vi "get_ACS_status.vi"() -> ()   [LabVIEW 2018]
uses:
  S4GEI/S4GEI/RxTx/RxTx.lvclass
  <vilib>/addons/zeromq/socket_type.ctl
  <vilib>/addons/zeromq/socket_options.ctl
  <vilib>/addons/zeromq/zmq_socket.lvclass
  <vilib>/addons/zeromq/zmq_context.lvclass
  <vilib>/addons/zeromq/zeromq.lvlib
panel:
  in  "RxTx in":refnum<class "RxTx.lvclass">
  in  "Stop Button":bool
  out "error out":errorcluster
  out "error out 3":errorcluster
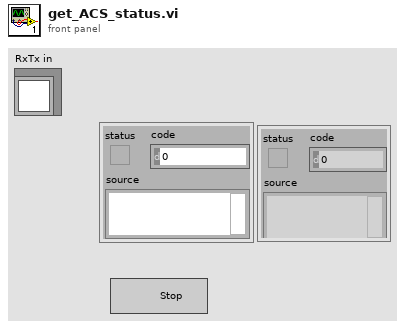
[diagram p1: front panel]
types:
  T1 = typedef "zeromq.lvlib/socket_options.ctl" = enum8{"NONE", "ZMQ_HWM", "<2>", "ZMQ_SWAP", "ZMQ_AFFINITY", "ZMQ_ROUTING_ID", "ZMQ_SUBSCRIBE", "ZMQ_UNSUBSCRIBE", "ZMQ_RATE", "ZMQ_RECOVERY_IVL", "ZMQ_MCAST_LOOP", "ZMQ_SNDBUF", "ZMQ_RCVBUF", "ZMQ_RCVMORE", "ZMQ_FD", "ZMQ_EVENTS", "ZMQ_TYPE", "ZMQ_LINGER", "ZMQ_RECONNECT_IVL", "ZMQ_BACKLOG", "ZMQ_RECOVERY_IVL_MSEC", "ZMQ_RECONNECT_IVL_MAX", "ZMQ_MAXMSGSIZE", "ZMQ_SNDHWM", "ZMQ_RCVHWM", "ZMQ_MULTICAST_HOPS", "<26>", "ZMQ_RCVTIMEO", "ZMQ_SNDTIMEO", "<29>", "<30>", "ZMQ_IPV4ONLY", "ZMQ_LAST_ENDPOINT", "ZMQ_ROUTER_MANDATORY", "ZMQ_TCP_KEEPALIVE", "ZMQ_TCP_KEEPALIVE_CNT", "ZMQ_TCP_KEEPALIVE_IDLE", "ZMQ_TCP_KEEPALIVE_INTVL", "ZMQ_TCP_ACCEPT_FILTER", "ZMQ_IMMEDIATE", "ZMQ_XPUB_VERBOSE", "ZMQ_ROUTER_RAW", "ZMQ_IPV6", "ZMQ_MECHANISM", "ZMQ_PLAIN_SERVER", "ZMQ_PLAIN_USERNAME", "ZMQ_PLAIN_PASSWORD", "ZMQ_CURVE_SERVER", "ZMQ_CURVE_PUBLICKEY", "ZMQ_CURVE_SECRETKEY", "ZMQ_CURVE_SERVERKEY", "ZMQ_PROBE_ROUTER", "ZMQ_REQ_CORRELATE", "ZMQ_REQ_RELAXED", "ZMQ_CONFLATE", "ZMQ_ZAP_DOMAIN", "ZMQ_ROUTER_HANDOVER", "ZMQ_TOS", "ZMQ_IPC_FILTER_PID", "ZMQ_IPC_FILTER_UID", "ZMQ_IPC_FILTER_GID", "ZMQ_CONNECT_ROUTING_ID", "ZMQ_GSSAPI_SERVER", "ZMQ_GSSAPI_PRINCIPAL", "ZMQ_GSSAPI_SERVICE_PRINCIPAL", "ZMQ_GSSAPI_PLAINTEXT", "ZMQ_HANDSHAKE_IVL", "<67>", "ZMQ_SOCKS_PROXY", "ZMQ_XPUB_NODROP", "ZMQ_BLOCKY", "ZMQ_XPUB_MANUAL", "ZMQ_XPUB_WELCOME_MSG", "ZMQ_STREAM_NOTIFY", "ZMQ_INVERT_MATCHING", "ZMQ_HEARTBEAT_IVL", "ZMQ_HEARTBEAT_TTL", "ZMQ_HEARTBEAT_TIMEOUT", "ZMQ_XPUB_VERBOSER", "ZMQ_CONNECT_TIMEOUT", "ZMQ_TCP_MAXRT", "ZMQ_THREAD_SAFE", "<82>", "<83>", "ZMQ_MULTICAST_MAXTPDU", "ZMQ_VMCI_BUFFER_SIZE", "ZMQ_VMCI_BUFFER_MIN_SIZE", "ZMQ_VMCI_BUFFER_MAX_SIZE", "ZMQ_VMCI_CONNECT_TIMEOUT", "ZMQ_USE_FD", "ZMQ_GSSAPI_PRINCIPAL_NAMETYPE", "ZMQ_GSSAPI_SERVICE_PRINCIPAL_NAMETYPE", "ZMQ_BINDTODEVICE", "ZMQ_ZAP_ENFORCE_DOMAIN", "ZMQ_LOOPBACK_FASTPATH", "ZMQ_METADATA", "ZMQ_MULTICAST_LOOP", "ZMQ_ROUTER_NOTIFY"}
  T2 = typedef "zeromq.lvlib/socket_type.ctl" = enum8{"ZMQ_PAIR", "ZMQ_PUB", "ZMQ_SUB", "ZMQ_REQ", "ZMQ_REP", "ZMQ_DEALER", "ZMQ_ROUTER", "ZMQ_PULL", "ZMQ_PUSH", "ZMQ_XPUB", "ZMQ_XSUB", "ZMQ_STREAM", "ZMQ_SERVER", "ZMQ_CLIENT", "ZMQ_RADIO", "ZMQ_DISH", "ZMQ_GATHER", "ZMQ_SCATTER", "ZMQ_DGRAM"}
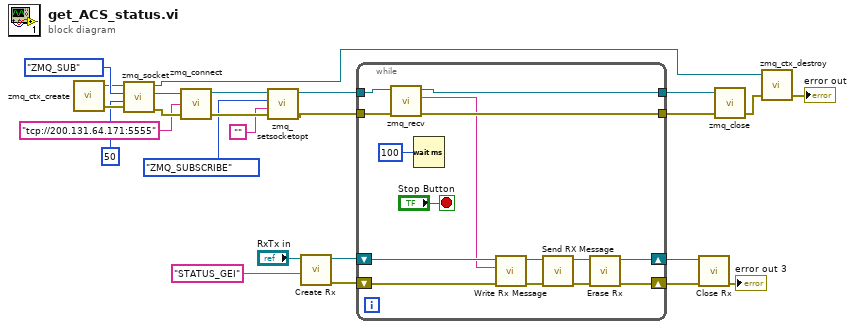
[diagram p0: block diagram]
diagram:
  n1 = call <vilib>:"zmq_ctx_create.vi"() -> ("error out"=w13:errorcluster, "context out"=w5:refnum<class "zmq_context.lvclass">)  [unwired: 4 in]
  n2 = call <vilib>:"zmq_socket.vi"("error in"=w13, "linger (ms)"=50, "socket type"=socket_type."ZMQ_SUB", "context in"=w5) -> ("error out"=w12:errorcluster, "socket out"=w6:refnum<class "zmq_socket.lvclass">, "context out"=w1:refnum<class "zmq_context.lvclass">)  [unwired: 1 in]
  n3 = call <vilib>:"zmq_connect.vi"("error in"=w12, "endpoint"="tcp://200.131.64.171:5555", "socket in"=w6) -> ("error out"=w10:errorcluster, "socket out"=w11:refnum<class "zmq_socket.lvclass">)  [unwired: 1 in]
  n4 = call <vilib>:"zmq_setsocketopt.vi"("error in"=w10, "value"="", "option"=socket_options."ZMQ_SUBSCRIBE", "socket in"=w11) -> ("error out"=w3:errorcluster, "socket out"=w2:refnum<class "zmq_socket.lvclass">)  [unwired: 2 in]
  n5 = call "Create Rx.vi"("Reader Name"="STATUS_GEI" ("Writer Name"), "RxTx in"="RxTx in") -> ("error out"=w19:errorcluster, "RxTx out"=w20:refnum<class "RxTx.lvclass">)  [unwired: 8 in]
  n6 = while {
    shift-right: [w34] -> w18
    shift-left: w20 -> [w27]
    shift-right: [w33] -> w17
    shift-left: w19 -> [w28]
    tunnel: w2 -> [w39]
    tunnel: w3 -> [w38]
    tunnel: [w37] -> w24
    tunnel: [w36] -> w23
    stop <- "Stop Button" stop-if-true
    n7 = call <vilib>:"zmq_recv.vi"("error in"=w38, "socket in"=w39) -> ("error out"=w36:errorcluster, "data"=w26:string, "socket out"=w37:refnum<class "zmq_socket.lvclass">)  [unwired: 3 in, 2 out]
    n8 = Wait (ms)(milliseconds to wait=u32 100) -> ()  [unwired: 1 out]
    n9 = call "Write Rx Message.vi"("error in (no error)"=w28, "Rx Message"=w26, "RxTx in"=w27) -> ("error out"=w29:errorcluster, "RxTx out"=w30:refnum<class "RxTx.lvclass">)  [unwired: 7 in]
    n10 = call "Send RX Message.vi"("error in (no error)"=w29, "RxTx in"=w30) -> ("error out"=w32:errorcluster, "RxTx out"=w35:refnum<class "RxTx.lvclass">)  [unwired: 8 in]
    n11 = call "Erase Rx.vi"("error in (no error)"=w32, "RxTx in"=w35) -> ("error out"=w33:errorcluster, "RxTx out"=w34:refnum<class "RxTx.lvclass">)  [unwired: 8 in]
  }
  n12 = call "Close Rx.vi"("error in (no error)"=w17, "RxTx in"=w18) -> ("error out"=→"error out 3":errorcluster)  [unwired: 8 in, 1 out]
  n13 = call <vilib>:"zmq_close.vi"("error in"=w23, "socket"=w24) -> ("error out"=w25:errorcluster)  [unwired: 3 in]
  n14 = call <vilib>:"zmq_ctx_destroy.vi"("error in"=w25, "context in"=w1) -> ("error out"=→"error out":errorcluster)  [unwired: 3 in]
